vi "Update.vi"(10 "Y":dbl, 11 "LinealFitting in":refnum<class "LinealFitting.lvclass">) -> (3 "LinealFitting out":refnum<class "LinealFitting.lvclass">)   [LabVIEW 2019, in "LinealFitting.lvclass"]
uses:
  LinealFitting.lvclass
  LinealFitting.lvclass/LinealFitting.ctl
  <vilib>/Analysis/NI_AALPro.lvlib
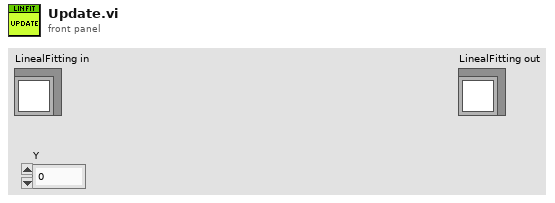
[diagram p1: front panel]
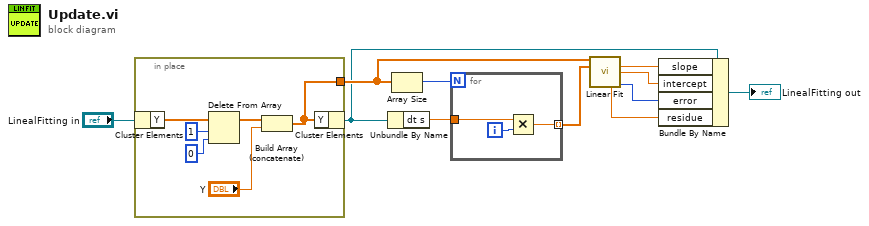
[diagram p0: block diagram]
diagram:
  n1 = in-place {
    in-place-border: [w12] -> w7
    n2 = in-place-cluster #1("LinealFitting in") -> ("Y"=w17:dbl[])
    n3 = Delete From Array(array=w17, length=1, index=0) -> (array with subset deleted=w14:dbl[])  [unwired: 1 out]
    n4 = Build Array (concatenate)(w14, "Y") -> (w12:dbl[])
    n5 = in-place-cluster #1("Y"=w12) -> (w6:refnum<class "LinealFitting.lvclass">)
  }
  n6 = Unbundle By Name(w6) -> ("dt s"=w10:dbl)
  n7 = Array Size(array=w7) -> (size(s)=w9:i32)
  n8 = for {
    N: w9 -> [_]
    tunnel: w10 -> [w19]
    tunnel: [w18] -> w8 mode=indexing
    i -> [w20]
    n9 = Multiply(x=w19, y=w20) -> (x*y=w18:dbl)
  }
  n10 = call <vilib>:"Linear Fit.vi"("Y"=w7, "X"=w8) -> ("slope"=w5:dbl, "intercept"=w4:dbl, "residue"=w3:dbl, "error"=w1:i32)  [unwired: 9 in, 1 out]
  n11 = Bundle By Name(cluster=w6, "slope"=w5, "intercept"=w4, "error"=w1, "residue"=w3) -> (→"LinealFitting out":refnum<class "LinealFitting.lvclass">)
